vi "Read New Delimiters.vi"(8 "Error In":errorcluster, 11 "SetDelimiter In":refnum<class "SetDelimiter.lvclass">) -> (0 "Error Out":errorcluster, 2 "New Delimiters":cluster{"Close":string, "Open":string}, 3 "SetDelimiter Out":refnum<class "SetDelimiter.lvclass">)   [LabVIEW 2018, in "Toolkit.lvlib" / "Tokens.lvlib" / "SetDelimiter.lvclass"]
uses:
  SetDelimiter.lvclass
  SetDelimiter.lvclass/SetDelimiter.ctl
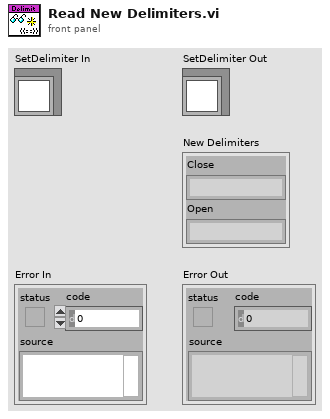
[diagram p1: front panel]
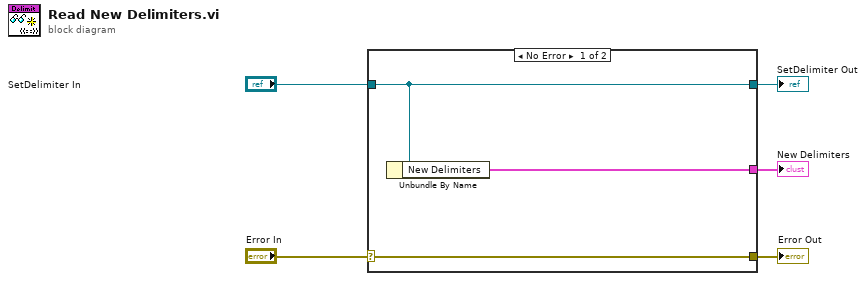
[diagram p0: block diagram]
diagram:
  n1 = case shown="No Error" "Error In" {
    selector: "Error In" -> [w8 w9]
    tunnel: [w8 w9] -> w4
    tunnel: [w7 w10] -> w2
    tunnel: "SetDelimiter In" -> [w7 w10]
    tunnel: [w6 _] -> w1
    frame No Error {
      n2 = Unbundle By Name(w7) -> ("New Delimiters"=w6:cluster{"Close":string, "Open":string})
    }
    frame Error {
    }
  }
  "Error Out" <- w4
  "SetDelimiter Out" <- w2
  "New Delimiters" <- w1
